vi "Command.Diagnostic Data Lookup Table Initialize.vi"(8 "error in (no error)":errorcluster, 11 "Command Refs":T1) -> (0 "error out":errorcluster {"code" min=0 max=0}, 3 "Diag Data Ref":T2)   [LabVIEW 2015, in "J1939 Addon Engine.lvlib"]
uses:
  J1939 Addon Engine.lvlib
  Types/Command.Diagnostic Data Lookup Table Reference.ctl
  Types/Command.Diagnostic Data Lookup Table State Variables.ctl
  Types/Command.Configuration.ctl
  Types/Command.Diagnostic Data Lookup Table Action.ctl
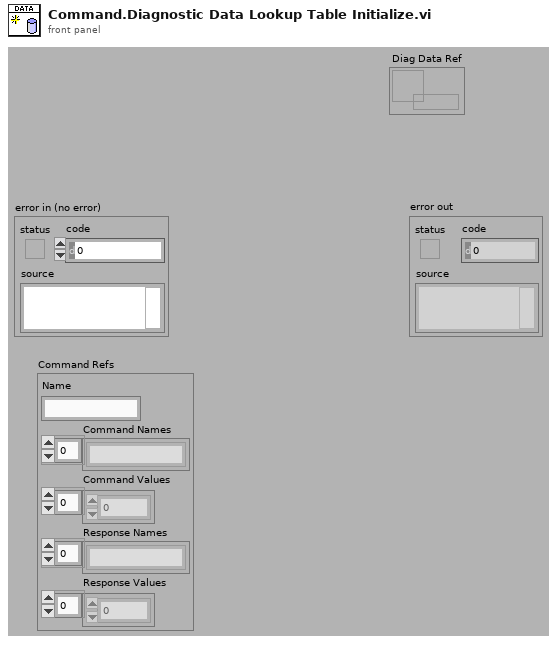
[diagram p1: front panel]
types:
  T1 = typedef "J1939 Addon Engine.lvlib/Command.Configuration.ctl" = cluster{"Name":string, "Command Names":string[], "Command Values":dbl[], "Response Names":string[], "Response Values":dbl[]}
  T2 = typedef "J1939 Addon Engine.lvlib/Command.Diagnostic Data Lookup Table Reference.ctl" = refnum<data-value>
  T3 = typedef "J1939 Addon Engine.lvlib/Command.Diagnostic Data Lookup Table State Variables.ctl" = cluster{"LUT":variant, "Response Names":string[], "Command Names":string[]}
  T4 = typedef "J1939 Addon Engine.lvlib/Command.Diagnostic Data Lookup Table Action.ctl" = enum16{"Initialize", "Get All", "Set All", "Set Value", "Get Value"}
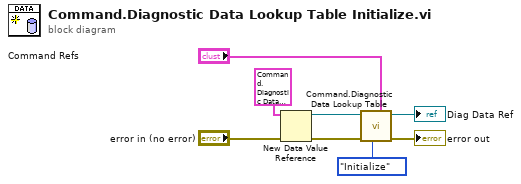
[diagram p0: block diagram]
diagram:
  n1 = New Data Value Reference(data value=T3 {"LUT"=variant, "Response Names"=[], "Command Names"=[]}, error in="error in (no error)") -> (data value reference=w3:refnum<data-value>, error out=w2:errorcluster)
  n2 = call "Command.Diagnostic Data Lookup Table.vi"("Command Refs"="Command Refs", "command"=Command.Diagnostic_Data_Lookup_Table_Action."Initialize", "error in (no error)"=w2, "Diag Data Ref"=w3) -> ("error out"=→"error out":errorcluster, "Diag Data Ref out"=→"Diag Data Ref":T2)  [unwired: 4 in, 2 out]
